vi "Actor Core.vi"(8 "error in":errorcluster, 11 "Prime Panel in":refnum<class "Configuration Editor.lvclass">) -> (0 "error out":errorcluster, 3 "Actor out":refnum<class "Actor.lvclass">)   [LabVIEW 2023, in "Configuration Editor.lvlib" / "Configuration Editor.lvclass"]
doc: "Base class for the <b>Prime</b> subpanel.\nThis provides the basic implementation for show/hide operations.\n\nancestor classes should override this, but maintain proportions."
uses:
  Library/Configuration Editor.lvclass
  builds/Framework/Actor Framework.lvlibp/1abvi3w/vi.lib/ActorFramework/Actor/Actor.lvclass
  Configuration Editor Messages/Select Device Msg/Select Device Msg.lvclass/Select Device Msg.ctl
  builds/Framework/Actor Framework.lvlibp/1abvi3w/vi.lib/ActorFramework/Message Enqueuer/Enqueue.vi
  Configuration Editor Messages/Add Device Msg/Add Device Msg.lvclass
  Configuration Editor Messages/Remove Device Msg/Remove Device Msg.lvclass
  Configuration Editor Messages/Select Device Msg/Select Device Msg.lvclass
  builds/Main/Docking.lvlibp/Prime Panel/PrimeDock.lvclass
  builds/Framework/Engine.lvlibp/Engine/Library/Engine.lvclass
  C:/Users/Public/Documents/Development/builds/Framework/Engine.lvlibp/Engine/Library/Engine.lvclass
panel:
  in  "Save":bool
  in  "Refresh":bool
  in  "Remove":bool
  in  "Add":bool
  in  "Signal List":i32(listbox)
  in  "Keys":i32(listbox)
  in  "Instruments":i32(listbox)
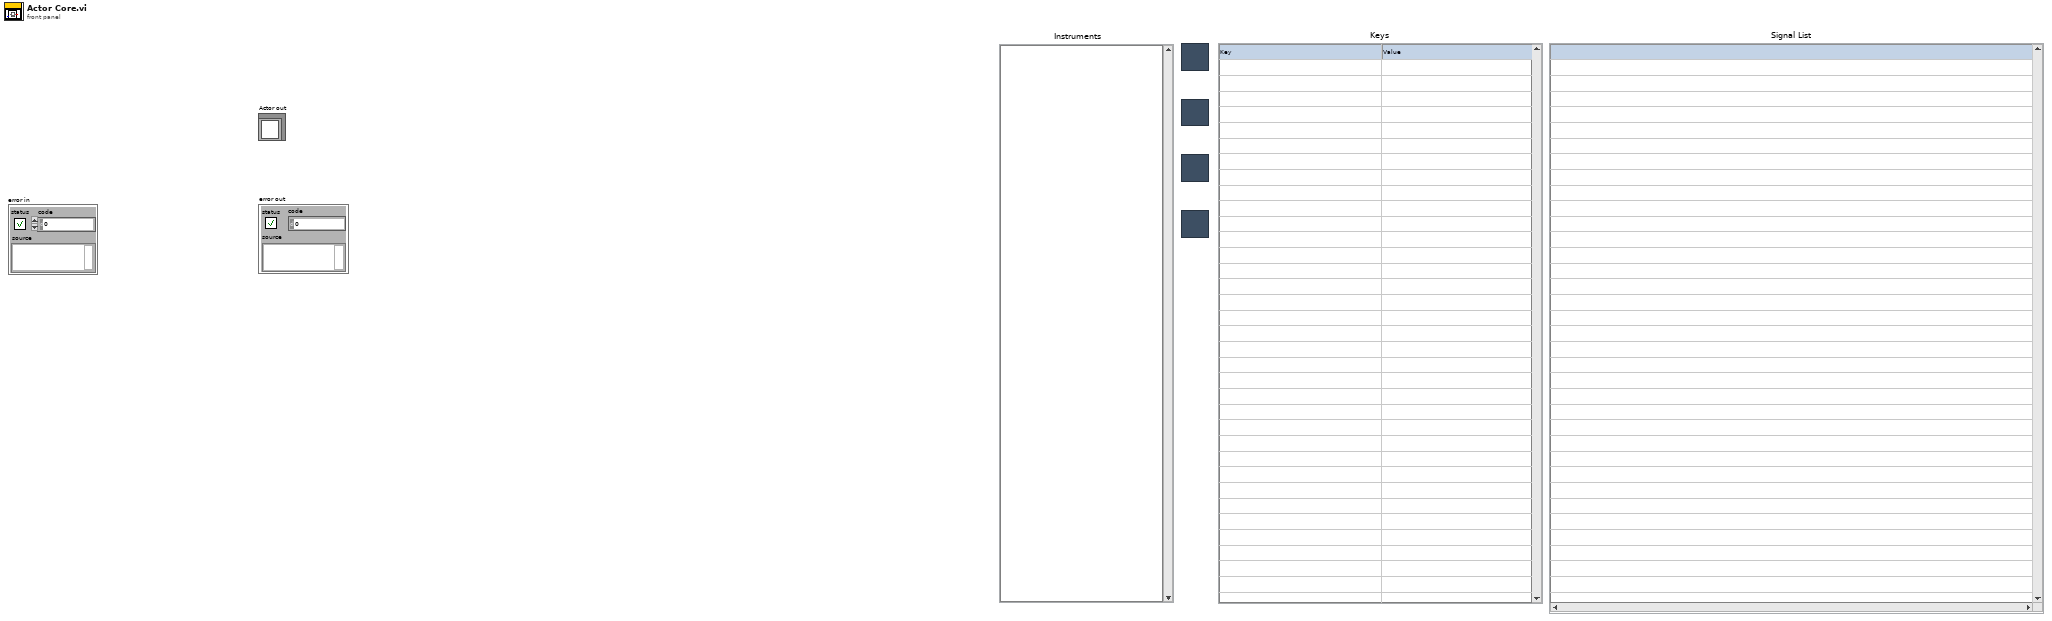
[diagram p1: front panel]
types:
  T1 = cluster{"Pnl Actor":refnum<event-registration>, "Event Registration Refnum":refnum<event-registration>}
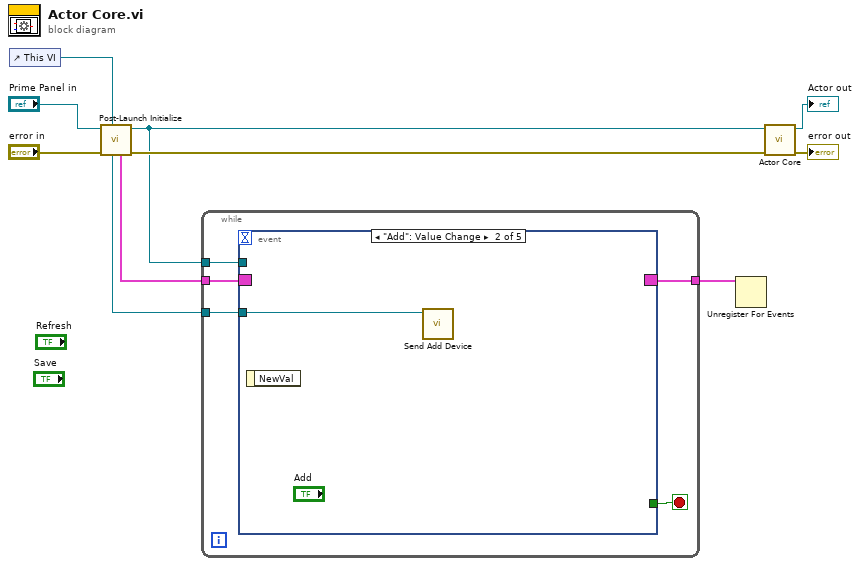
[diagram p0: block diagram]
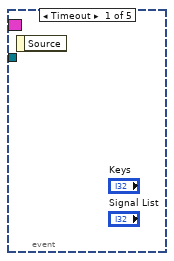
[diagram p2: hidden frame]
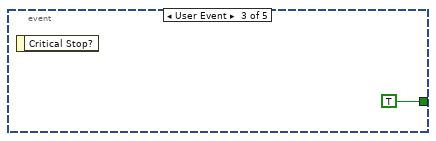
[diagram p3: hidden frame]
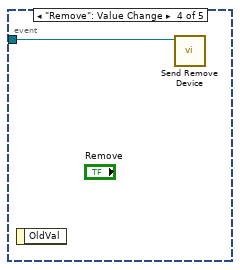
[diagram p4: hidden frame]
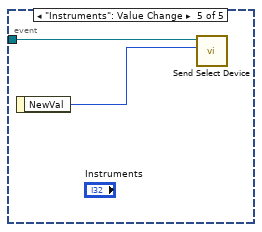
[diagram p5: hidden frame]
diagram:
  n1 = control-ref of="This VI"() -> (w5:refnum<vi>)
  n2 = call "Post-Launch Initialize.vi"("GUI Reference"=w5, "error in (no error)"="error in", "Engine in"="Prime Panel in") -> ("error out"=w6:errorcluster, "Engine out"=w2:refnum<class "Configuration Editor.lvclass">, "Registered Events"=w4:T1, "Self Enqueuer"=w3:refnum<class "Message Enqueuer.lvclass">)  [unwired: 5 in]
  n3 = while {
    tunnel: w4 -> [w15]
    tunnel: w3 -> [w14]
    tunnel: w2 -> [w13]
    tunnel: [w12] -> w1
    stop <- w11 stop-if-true
    n4 = event shown="[1] \"Add\": Value Change" {
      selector: w15 -> [_ _ _ _ _]
      dyn-events: [_ _ _ _ _] -> w12
      timeout: _ -> [_ _ _ _ _]
      tunnel: w14 -> [_ w16 _ w18 w20]
      tunnel: w13 -> [_ _ _ _ _]
      tunnel: [_ _ TRUE _ _] -> w11
      event Timeout {
        n5 = event-data() -> ()  [unwired: 1 in, 1 out]
      }
      event "Add": Value Change {
        n6 = event-data() -> ()  [unwired: 1 in, 1 out]
        n7 = call "Send Add Device.vi"("Message Enqueuer"=w16) -> ()  [unwired: 9 in, 2 out]
      }
      event User Event {
        n8 = event-data() -> ()  [unwired: 1 in, 1 out]
      }
      event "Remove": Value Change {
        n9 = event-data() -> ()  [unwired: 1 in, 1 out]
        n10 = call "Send Remove Device.vi"("Message Enqueuer"=w18) -> ()  [unwired: 9 in, 2 out]
      }
      event "Instruments": Value Change {
        n11 = event-data() -> ("NewVal"=w19:i32)  [unwired: 1 in]
        n12 = call "Send Select Device.vi"("Selected"=w19, "Message Enqueuer"=w20) -> ()  [unwired: 8 in, 2 out]
      }
    }
  }
  n13 = Unregister For Events(event registration refnum=w1) -> ()  [unwired: 1 in, 1 out]
  n14 = call-parent "Actor Core.vi"("error in"=w6, "Prime Panel in"=w2) -> ("error out"=→"error out":errorcluster, "Actor out"=→"Actor out":refnum<class "Actor.lvclass">)  [unwired: 8 in]
